vi "Create Command.vi"(5 "Invert Condition (F)":bool, 7 "Condition":T2, 8 "error in (no error)":errorcluster, 11 "Op Code":T1) -> (0 "error out":errorcluster, 2 "Instruction":u16 format="%016b")   [LabVIEW 2020, in "BCI-1553 API.lvlib"]
doc: "Creates an instruction list command. A command is made up of an Op Code and Condition that are concatenated in a single U16. For full range of operation, the condition may be inverted."
uses:
  BCI-1553 API.lvlib
  TypeDefs/BC Condition Codes.ctl
  TypeDefs/BC Op Codes - Verbose.ctl
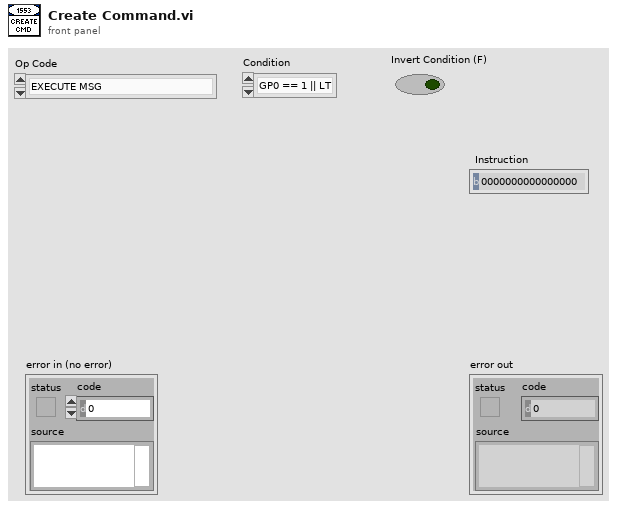
[diagram p1: front panel]
types:
  T1 = typedef "BCI-1553 API.lvlib/BC Op Codes - Verbose.ctl" = enum16{"EXECUTE MSG", "EXECUTE MSG GO", "JUMP", "CALL SUBROUTINE", "RETURN", "INTERRUPT REQUEST", "HALT", "DELAY", "WAIT FRAME TIMER = 0", "COMPARE FRAME TIMER", "COMPARE MSG TIMER", "LOAD TIME TAG CTR", "LOAD TIME TAG CTR HI", "LOAD FRAME TIMER", "START FRAME TIMER", "PUSH TIME TAG COUNT", "PUSH TIME TAG COUNT HI", "PUSH TIME TAG COUNT BOTH", "PUSH BLOCK STATUS WORD", "PUSH CURRENT VALUE", "PUSH INDIRECT", "WAIT EXT TRIGGER", "EXECUTE AND FLIP", "EXECUTE, FLIP, GO", "WRITE VALUE TO WMI", "WRITE VALUE TO MEM", "DECREMENT RAM, SKIP", "FLAG"}
  T2 = typedef "BCI-1553 API.lvlib/BC Condition Codes.ctl" = enum16{"GP0 == 1 || LT", "GP1 == 1 || NE", "GP2 == 1", "GP3 == 1", "GP4 == 1", "GP5 == 1", "GP6 == 1", "GP7 == 1", "NORESP", "FMTERR", "GOODBLOCK", "MSKSTATSET", "BADMSG", "1RETRY", "2RETRY", "ALWAYS"}
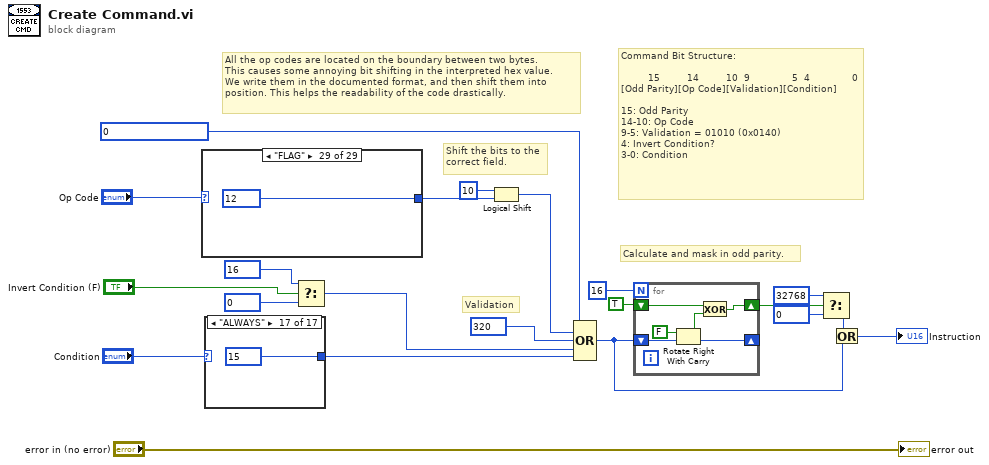
[diagram p0: block diagram]
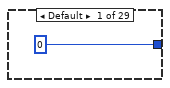
[diagram p2: hidden frame]
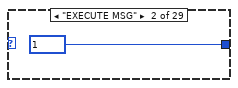
[diagram p3: hidden frame]
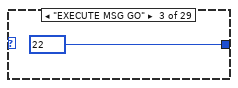
[diagram p4: hidden frame]
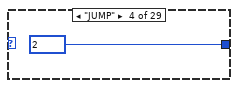
[diagram p5: hidden frame]
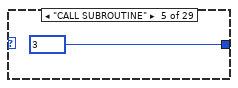
[diagram p6: hidden frame]
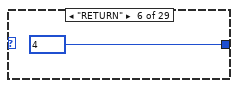
[diagram p7: hidden frame]
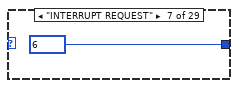
[diagram p8: hidden frame]
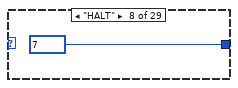
[diagram p9: hidden frame]
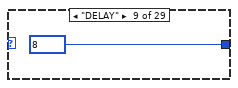
[diagram p10: hidden frame]
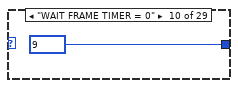
[diagram p11: hidden frame]
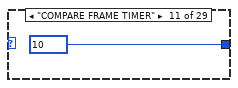
[diagram p12: hidden frame]
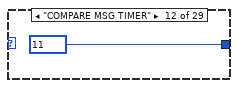
[diagram p13: hidden frame]
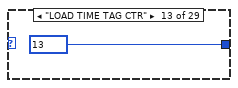
[diagram p14: hidden frame]
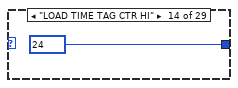
[diagram p15: hidden frame]
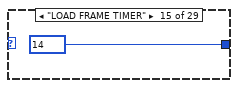
[diagram p16: hidden frame]
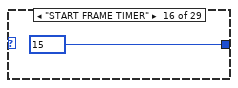
[diagram p17: hidden frame]
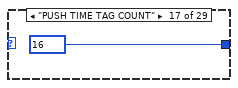
[diagram p18: hidden frame]
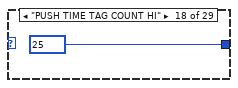
[diagram p19: hidden frame]
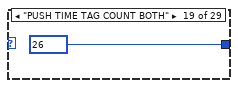
[diagram p20: hidden frame]
diagram:
  # "Shift the bits to the\ncorrect field."
  # "All the op codes are located on the boundary between two bytes.\nThis causes some annoying bit shifting in the interpreted hex value.\nWe write them in the documented format, and then shift them into\nposition. This helps the readability of the code drastically."
  # "Calculate and mask in odd parity."
  # "Validation"
  # "Command Bit Structure:\n\n         15         14         10  9              5  4              0\n[Odd Parity][Op Code][Validation][Condition]\n\n15: Odd Parity\n14-10: Op Code\n9-5: Validation = 01010 (0x0140)\n4: Invert Condition?\n3-0: Condition"
  n1 = case shown="\"FLAG\"" "Op Code" {
    tunnel: [u16 0 u16 1 u16 22 u16 2 u16 3 u16 4 u16 6 u16 7 u16 8 u16 9 u16 10 u16 11 u16 13 u16 24 u16 14 u16 15 u16 16 u16 25 u16 26 u16 17 u16 18 u16 19 u16 20 u16 21 u16 23 u16 27 u16 28 u16 29 u16 12] -> w10
    frame Default {
    }
    frame "EXECUTE MSG" {
    }
    frame "EXECUTE MSG GO" {
    }
    frame "JUMP" {
    }
    frame "CALL SUBROUTINE" {
    }
    frame "RETURN" {
    }
    frame "INTERRUPT REQUEST" {
    }
    frame "HALT" {
    }
    frame "DELAY" {
    }
    frame "WAIT FRAME TIMER = 0" {
    }
    frame "COMPARE FRAME TIMER" {
    }
    frame "COMPARE MSG TIMER" {
    }
    frame "LOAD TIME TAG CTR" {
    }
    frame "LOAD TIME TAG CTR HI" {
    }
    frame "LOAD FRAME TIMER" {
    }
    frame "START FRAME TIMER" {
    }
    frame "PUSH TIME TAG COUNT" {
    }
    frame "PUSH TIME TAG COUNT HI" {
    }
    frame "PUSH TIME TAG COUNT BOTH" {
    }
    frame "PUSH BLOCK STATUS WORD" {
    }
    frame "PUSH CURRENT VALUE" {
    }
    frame "PUSH INDIRECT" {
    }
    frame "WAIT EXT TRIGGER" {
    }
    frame "EXECUTE AND FLIP" {
    }
    frame "EXECUTE, FLIP, GO" {
    }
    frame "WRITE VALUE TO WMI" {
    }
    frame "WRITE VALUE TO MEM" {
    }
    frame "DECREMENT RAM, SKIP" {
    }
    frame "FLAG" {
    }
  }
  n2 = case shown="\"ALWAYS\"" "Condition" {
    tunnel: [u16 0 u16 0 u16 1 u16 2 u16 3 u16 4 u16 5 u16 6 u16 7 u16 8 u16 9 u16 10 u16 11 u16 12 u16 13 u16 14 u16 15] -> w19
    frame Default {
    }
    frame "GP0 == 1 || LT" {
    }
    frame "GP1 == 1 || NE" {
    }
    frame "GP2 == 1" {
    }
    frame "GP3 == 1" {
    }
    frame "GP4 == 1" {
    }
    frame "GP5 == 1" {
    }
    frame "GP6 == 1" {
    }
    frame "GP7 == 1" {
    }
    frame "NORESP" {
    }
    frame "FMTERR" {
    }
    frame "GOODBLOCK" {
    }
    frame "MSKSTATSET" {
    }
    frame "BADMSG" {
    }
    frame "1RETRY" {
    }
    frame "2RETRY" {
    }
    frame "ALWAYS" {
    }
  }
  n3 = Select(t=u16 16, s="Invert Condition (F)", f=u16 0) -> (s? t:f=w14:u16)
  n4 = Logical Shift(y=i16 10, x=w10) -> (x << y=w11:u16)
  n5 = Compound Arithmetic op=OR(u16 0, w11, u16 320, w14, w19) -> (w2:u16)
  n6 = for {
    N: 16 -> [_]
    shift-right: [w72] -> _
    shift-left: w2 -> [w73]
    shift-right: [w68] -> w6
    shift-left: TRUE -> [w69]
    n7 = Rotate Right With Carry(2:w73, 3:FALSE ("carry")) -> (0:w72:u16, 1:w70:bool)
    n8 = Exclusive Or(1:w70, 2:w69) -> (0:w68:bool)
  }
  n9 = Select(t=u16 32768, s=w6, f=u16 0) -> (s? t:f=w3:u16)
  n10 = Or(x=w3, y=w2) -> (x .or. y?=→"Instruction":u16)
  "error out" <- "error in (no error)"
